vi "InitializeVariables.vi"() -> (3 "InitializeCluster":T1)   [LabVIEW 2013]
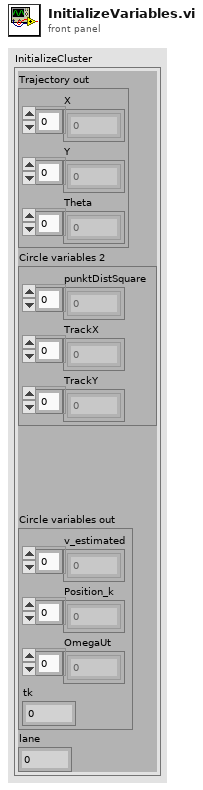
[diagram p1: front panel]
types:
  T1 = cluster{"Trajectory out":cluster{"X":dbl[], "Y":dbl[], "Theta":dbl[]}, "Circle variables 2":cluster{"punktDistSquare":cdb[], "TrackX":dbl[], "TrackY":dbl[]}, "Circle variables out":cluster{"v_estimated":cdb[], "Position_k":dbl[], "OmegaUt":dbl[], "tk":dbl}, "lane":i32}
  T2 = cluster{"v_estimated":cdb[], "Position_k":dbl[], "OmegaUt":dbl[], "tk":dbl}
  T3 = cluster{"punktDistSquare":cdb[], "TrackX":dbl[], "TrackY":dbl[]}
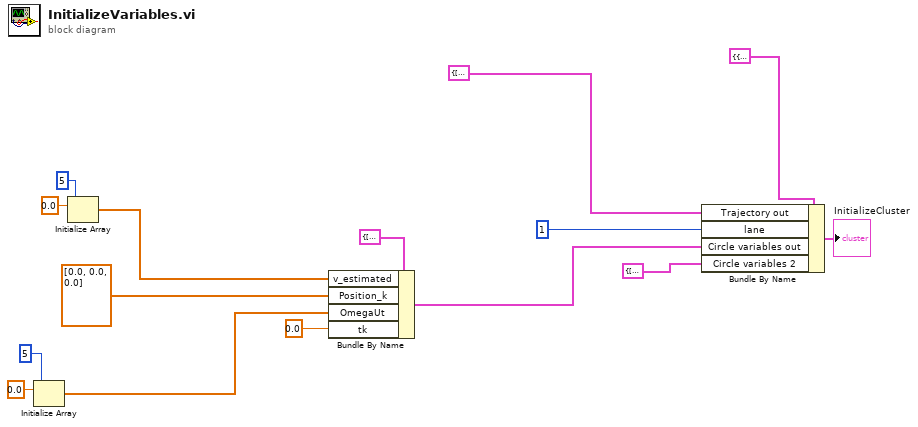
[diagram p0: block diagram]
diagram:
  n1 = Initialize Array(0.0 ("element"), 5 ("Number of values for median steering angle")) -> (w10:dbl[])
  n2 = Initialize Array(0.0 ("element"), 5 ("Number of values for median velocity")) -> (w11:dbl[])
  n3 = Bundle By Name(cluster=T2 {"v_estimated"=[], "Position_k"=[], "OmegaUt"=[], "tk"=0.0} ("Circle variables out"), "v_estimated"=w11, "Position_k"=dbl[] [0.0, 0.0, 0.0], "OmegaUt"=w10, "tk"=0.0 ("t0")) -> (w3:T2)
  n4 = Bundle By Name(cluster=T1 {"Trajectory out"={"X"=[], "Y"=[], "Theta"=[]}, "Circle variables 2"={"punktDistSquare"=[], "TrackX"=[], "TrackY"=[]}, "Circle variables out"={"v_estimated"=[], "Position_k"=[], "OmegaUt"=[], "tk"=0.0}, "lane"=0} ("Circle output"), "Trajectory out"=cluster{"X":dbl[], "Y":dbl[], "Theta":dbl[]} {"X"=[0.0], "Y"=[0.0], "Theta"=[0.0]}, "lane"=1 ("Starting lane"), "Circle variables out"=w3, "Circle variables 2"=T3 {"punktDistSquare"=[], "TrackX"=[], "TrackY"=[]}) -> (→"InitializeCluster":T1)
